vi "PI with FF.vi"(0 "Run PI?":bool, 1 "PIcluster":cluster{"SlewRate":dbl, "Kp":dbl, "Ki":dbl}, 2 "FFcluster":cluster{"FF_m":dbl, "FF_b":dbl}, 3 "LimitCluster":cluster{"Step":dbl, "CmdMax":dbl, "CmdMin":dbl}, 5 "SP":dbl, 7 "Error":dbl, 11 "RevCtrlZero":bool) -> (8 "Output":dbl)   [LabVIEW 2013]
uses:
  <vilib>/addons/control/pid/pid.llb/PID Output Rate Limiter (DBL).vi
  <vilib>/addons/control/pid/NI_PID_pid.lvlib
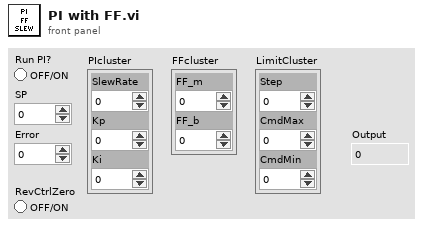
[diagram p1: front panel]
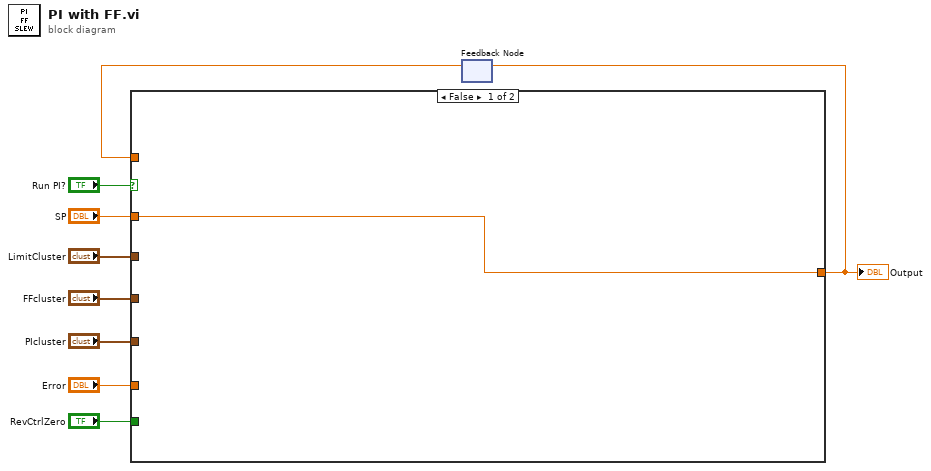
[diagram p0: block diagram]
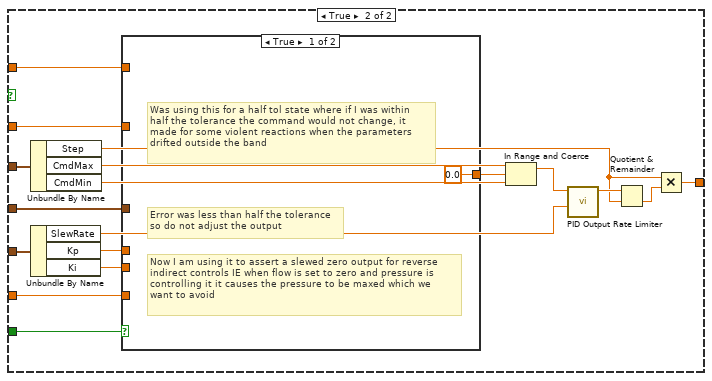
[diagram p2: hidden frame]
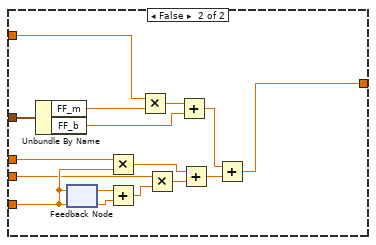
[diagram p3: hidden frame]
diagram:
  n1 = feedback #1() -> (w1:dbl)  [unwired: 1 in]
  n2 = case shown="False" "Run PI?" {
    tunnel: [w10 w15] -> w2
    tunnel: "SP" -> [w10 w28]
    tunnel: "Error" -> [_ w27]
    tunnel: "FFcluster" -> [_ w26]
    tunnel: "PIcluster" -> [_ w22]
    tunnel: "LimitCluster" -> [_ w23]
    tunnel: "RevCtrlZero" -> [_ w25]
    tunnel: w1 -> [_ w24]
    frame False {
    }
    frame True {
      n3 = Unbundle By Name(w23) -> ("Step"=w16:dbl, "CmdMax"=w12:dbl, "CmdMin"=w11:dbl)
      n4 = Unbundle By Name(w22) -> ("SlewRate"=w17:dbl, "Kp"=w21:dbl, "Ki"=w20:dbl)
      n5 = case shown="True" w25 {
        tunnel: w28 -> [_ w41]
        tunnel: w27 -> [_ w39]
        tunnel: w26 -> [_ w35]
        tunnel: w24 -> [_ _]
        tunnel: w21 -> [_ w32]
        tunnel: w20 -> [_ w31]
        tunnel: [0.0 ("CmdMax") w30] -> w14
        frame True {
          # "Now I am using it to assert a slewed zero output for reverse\nindirect controls IE when flow is set to zero and pressure is\ncontrolling it it causes the pressure to be maxed which we\nwant to avoid"
          # "Was using this for a half tol state where if I was within\nhalf the tolerance the command would not change, it\nmade for some violent reactions when the parameters\ndrifted outside the band"
          # "Error was less than half the tolerance\nso do not adjust the output"
        }
        frame False {
          n6 = Unbundle By Name(w35) -> ("FF_m"=w34:dbl, "FF_b"=w33:dbl)
          n7 = feedback #2(w39) -> (w40:dbl)
          n8 = feedback-in #2(w39) -> ()
          n9 = Multiply(x=w32, y=w39) -> (x*y=w37:dbl)
          n10 = Add(x=w40, y=w39) -> (x+y=w36:dbl)
          n11 = Multiply(x=w41, y=w34) -> (x*y=w44:dbl)
          n12 = Multiply(x=w31, y=w36) -> (x*y=w38:dbl)
          n13 = Add(x=w44, y=w33) -> (x+y=w43:dbl)
          n14 = Add(x=w37, y=w38) -> (x+y=w42:dbl)
          n15 = Add(x=w43, y=w42) -> (x+y=w30:dbl)
        }
      }
      n16 = In Range and Coerce(upper limit=w12, x=w14, lower limit=w11) -> (coerced(x)=w13:dbl)  [unwired: 1 out]
      n17 = call-poly <vilib>:"PID Output Rate Limiter.vi"("output rate (EGU/min)"=w17, "input (controller output)"=w13) -> ("output"=w19:dbl)  [unwired: 6 in, 1 out]
      n18 = Quotient & Remainder(x=w19, y=w16) -> (floor(x/y)=w18:dbl)  [unwired: 1 out]
      n19 = Multiply(x=w16, y=w18) -> (x*y=w15:dbl)
    }
  }
  "Output" <- w2
  n20 = feedback-in #1(w2) -> ()
